vi "Hi-Tec_conversions.vi"(0 "Input":dbl format="%.3f", 1 "Conversion":T3(ring), 2 "Release temp (deg C)":dbl format="%.2f", 3 "Atmos Pres (mbars)":dbl format="%.2f", 4 "Hi-Tec calib":T1={"Ref temp (deg C)"=0.0, "Ref Pres (mbars)"=0.0, "Density at calib conditions"=-0.0141, "Coefficients"=[], "Fit"=enum."Cubic Hermite Spline"} {"Coefficients" format="%.2f"; "Density at calib conditions" format="%.4f"; "Ref Pres (mbars)" format="%.2f"; "Ref temp (deg C)" format="%.2f"}) -> (6 "Output":dbl format="%.3f", 7 "Flowrate (kg/min)":dbl format="%.4f")   [LabVIEW 2022 SP3]
uses:
  Controls/Hi-Tec_calib.ctl
  Controls/Hi-Tec Fitting.ctl
  <vilib>/gmath/NI_Gmath.lvlib
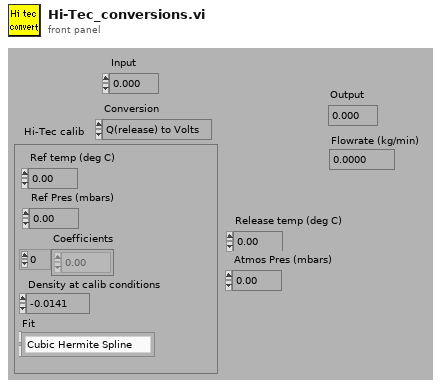
[diagram p1: front panel]
types:
  T1 = typedef "Hi-Tec_calib.ctl" = cluster{"Ref temp (deg C)":dbl, "Ref Pres (mbars)":dbl, "Density at calib conditions":dbl, "Coefficients":dbl[], "Fit":T2}
  T2 = typedef "Hi-Tec Fitting.ctl" = enum16{"Polynomial", "Cubic Hermite Spline"}
  T3 = enum16{"Q(release) to Volts", "Volts to Q(release)"}
  T4 = enum16{"Release to Reference", "Reference to Release"}
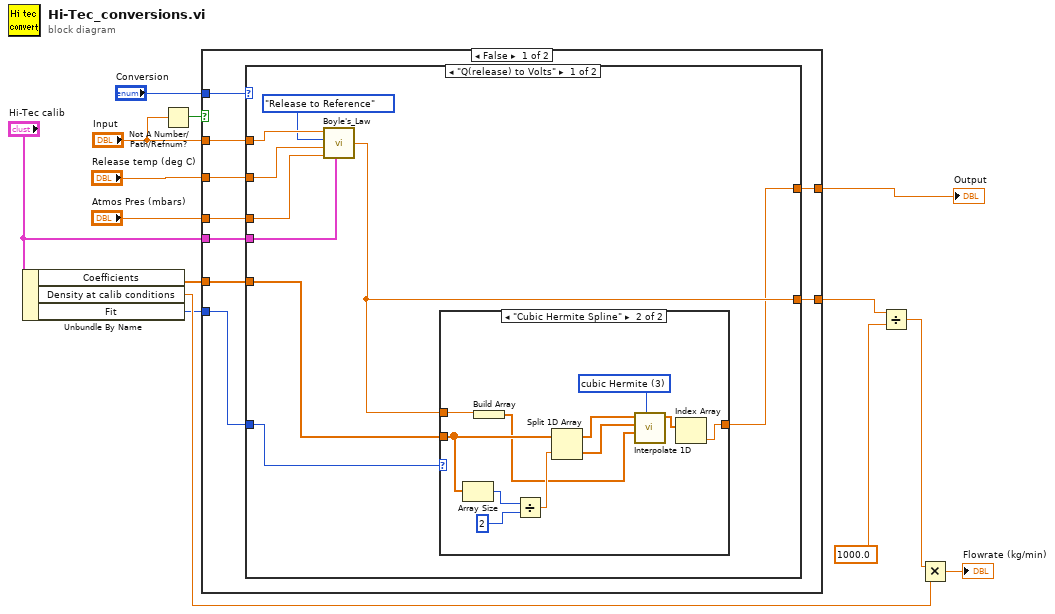
[diagram p0: block diagram]
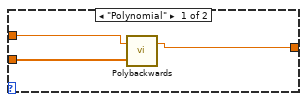
[diagram p2: hidden frame]
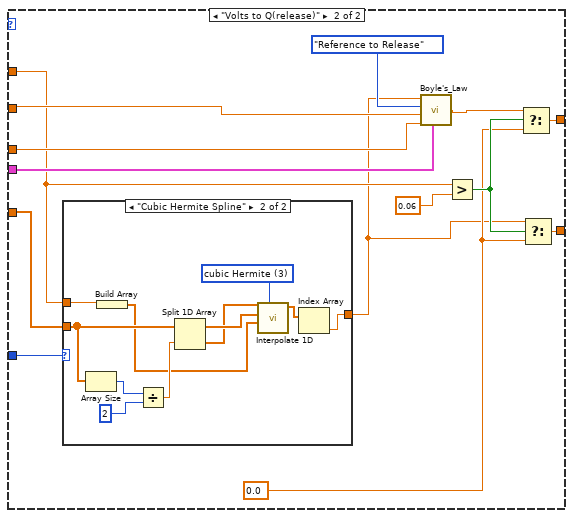
[diagram p3: hidden frame]
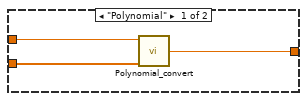
[diagram p4: hidden frame]
diagram:
  n1 = Unbundle By Name("Hi-Tec calib") -> ("Coefficients"=w13:dbl[], "Density at calib conditions"=w6:dbl, "Fit"=w1:T2)
  n2 = Not A Number/Path/Refnum?(number/path/refnum="Input") -> (NaN/Path/Refnum?=w2:bool)
  n3 = case shown="False" w2 {
    tunnel: "Conversion" -> [w23 _]
    tunnel: "Input" -> [w22 w75]
    tunnel: w13 -> [w21 _]
    tunnel: [w20 w75] -> w12
    tunnel: "Release temp (deg C)" -> [w19 _]
    tunnel: "Atmos Pres (mbars)" -> [w18 _]
    tunnel: "Hi-Tec calib" -> [w17 _]
    tunnel: [w16 w75] -> w4
    tunnel: w1 -> [w15 _]
    frame False {
      n4 = case shown="\"Q(release) to Volts\"" w23 {
        tunnel: w22 -> [w32 w50]
        tunnel: w21 -> [w26 w49]
        tunnel: [w24 w55] -> w20
        tunnel: w19 -> [w30 w58]
        tunnel: w18 -> [w29 w57]
        tunnel: w17 -> [w28 w59]
        tunnel: [w25 w53] -> w16
        tunnel: w15 -> [w27 w47]
        frame "Q(release) to Volts" {
          n5 = call "Boyle's_Law.vi"("Q in (l/min)"=w32, "Conversion"=T4."Release to Reference", "Release temp (deg C)"=w30, "Atmos Pres (mbars)"=w29, "Hi-Tec calib"=w28) -> ("Q out (l/min)"=w25:dbl)  [unwired: 2 out]
          n6 = case shown="\"Cubic Hermite Spline\"" w27 {
            tunnel: w25 -> [w34 w41]
            tunnel: w26 -> [w35 w43]
            tunnel: [w33 w39] -> w24
            frame "Polynomial" {
              n7 = call "Polybackwards.vi"("Coefficients"=w35, "Y input"=w34) -> ("X output"=w33:dbl)  [unwired: 1 out]
            }
            frame "Cubic Hermite Spline" {
              w46 = 3 items=["nearest", "linear", "spline", "cubic Hermite", "Lagrange"] ("method")
              n8 = Array Size(array=w43) -> (size(s)=w45:i32)
              n9 = Build Array(w41) -> (w40:dbl[])
              n10 = Divide(x=w45, y=2) -> (x/y=w42:dbl)
              n11 = Split 1D Array(array=w43, index=w42) -> (first subarray=w38:dbl[], second subarray=w37:dbl[])
              n12 = call <vilib>:"Interpolate 1D.vi"("method"=w46, "xi"=w40, "X"=w37, "Y"=w38) -> ("yi"=w36:dbl[])  [unwired: 5 in, 2 out]
              n13 = Index Array(array=w36) -> (element=w39:dbl)  [unwired: 1 in]
            }
          }
        }
        frame "Volts to Q(release)" {
          w52 = 0.0 ("f")
          n14 = case shown="\"Cubic Hermite Spline\"" w47 {
            tunnel: w50 -> [w63 w67]
            tunnel: w49 -> [w62 w71]
            tunnel: [w61 w65] -> w48
            frame "Polynomial" {
              n15 = call "Polynomial_convert.vi"("Calib constants"=w62, "Voltage"=w63) -> ("Eng Values"=w61:dbl)  [unwired: 4 out]
            }
            frame "Cubic Hermite Spline" {
              w74 = 3 items=["nearest", "linear", "spline", "cubic Hermite", "Lagrange"] ("method")
              n16 = Array Size(array=w71) -> (size(s)=w73:i32)
              n17 = Build Array(w67) -> (w66:dbl[])
              n18 = Divide(x=w73, y=2) -> (x/y=w70:dbl)
              n19 = Split 1D Array(array=w71, index=w70) -> (first subarray=w69:dbl[], second subarray=w68:dbl[])
              n20 = call <vilib>:"Interpolate 1D.vi"("method"=w74, "xi"=w66, "X"=w69, "Y"=w68) -> ("yi"=w64:dbl[])  [unwired: 5 in, 2 out]
              n21 = Index Array(array=w64) -> (element=w65:dbl)  [unwired: 1 in]
            }
          }
          n22 = call "Boyle's_Law.vi"("Q in (l/min)"=w48, "Conversion"=T4."Reference to Release", "Release temp (deg C)"=w58, "Atmos Pres (mbars)"=w57, "Hi-Tec calib"=w59) -> ("Q out (l/min)"=w56:dbl)  [unwired: 2 out]
          n23 = Greater?(x=w50, y=0.06) -> (0:w54:bool)
          n24 = Select(t=w56, s=w54, f=w52) -> (s? t:f=w55:dbl)
          n25 = Select(t=w48, s=w54, f=w52) -> (s? t:f=w53:dbl)
        }
      }
    }
    frame True {
    }
  }
  "Output" <- w12
  n26 = Divide(x=w4, y=1000.0) -> (x/y=w7:dbl)
  n27 = Multiply(x=w7, y=w6) -> (x*y=→"Flowrate (kg/min)":dbl)
